vi "RT_MATH_MovAvg.vi"(9 "Data_In":sgl, 10 "Sample_No":i32, 11 "Array_In":sgl[](array[numeric])) -> (2 "Data_Out":sgl, 3 "Array_Out":sgl[](array[numeric]))   [LabVIEW 2024]
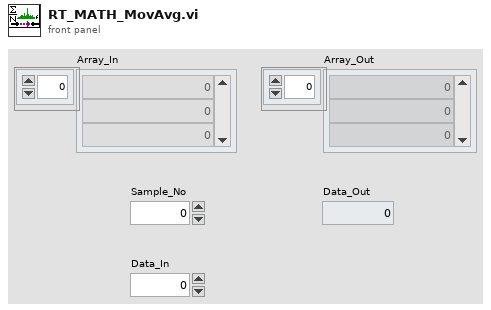
[diagram p1: front panel]
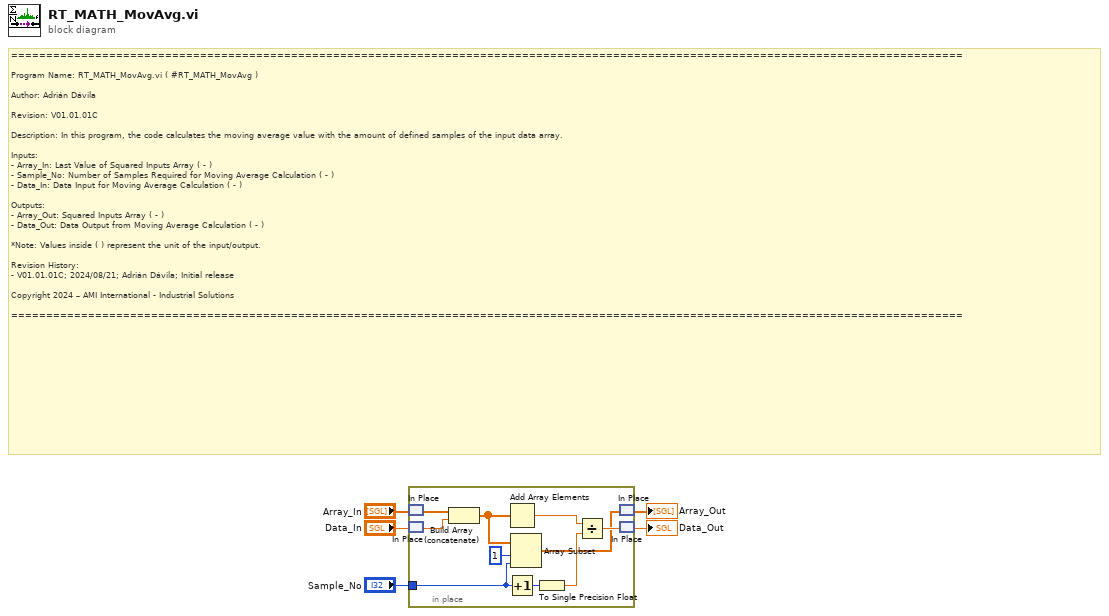
[diagram p0: block diagram]
diagram:
  # "========================================================================================================================================\n\nProgram Name: RT_MATH_MovAvg.vi ( #RT_MATH_MovAvg )\n\nAuthor: Adrián Dávila\n\nRevision: V01.01.01C\n\nDescription: In this program, the code calculates the moving average value with the amount of defined samples of the input data array. \n\nInputs:\n- Array_In: Last Value of Squared Inputs Array ( - )\n- Sample_No: Number of Samples Required for Moving Average Calculation ( - )\n- Data_In: Data Input for Moving Average Calculation ( - )\n\nOutputs:\n- Array_Out: Squared Inputs Array ( - )\n- Data_Out: Data Output from Moving Average Calculation ( - )\n\n*Note: Values inside ( ) represent the unit of the input/output.\n \nRevision History:\n- V01.01.01C; 2024/08/21; Adrián Dávila; Initial release\n\nCopyright 2024 – AMI International - Industrial Solutions\n\n========================================================================================================================================"
  n1 = in-place {
    in-place-border: "Sample_No" -> [w6]
    n2 = in-place-match #1("Array_In") -> (w10:sgl[])
    n3 = in-place-match #2("Data_In") -> (w9:sgl)
    n4 = Build Array (concatenate)(w10, w9) -> (w15:sgl[])
    n5 = Add Array Elements(numeric array=w15) -> (sum=w11:sgl)
    n6 = Increment(x=w6) -> (x+1=w14:i32)
    n7 = Array Subset(array=w15, index=1, length=w6) -> (w7:sgl[])
    n8 = To Single Precision Float(number=w14) -> (single precision float=w12:sgl)
    n9 = Divide(x=w11, y=w12) -> (x/y=w8:sgl)
    n10 = in-place-match #1(w7) -> (→"Array_Out":sgl[])
    n11 = in-place-match #2(w8) -> (→"Data_Out":sgl)
  }
